vi "set_iterations_per_pixel.vi"(8 "error in (no error)":errorcluster, 10 "iterations per pixel":i32, 11 "FPGAWrapperMH120124FrameScan_PXI7813R in":refnum<class "FPGAWrapperMH120124FrameScan_PXI7813R.lvclass">) -> (0 "error out":errorcluster, 3 "FPGAWrapperMH120124FrameScan_PXI7813R out":refnum<class "FPGAWrapperMH120124FrameScan_PXI7813R.lvclass">)   [LabVIEW 2010, in "FPGAWrapperMH120124FrameScan_PXI7813R.lvclass"]
uses:
  FPGAWrapperMH120124FrameScan_PXI7813R.lvclass
  FPGAWrapperMH120124FrameScan_PXI7813R.lvclass/FPGAWrapperMH120124FrameScan_PXI7813R.ctl
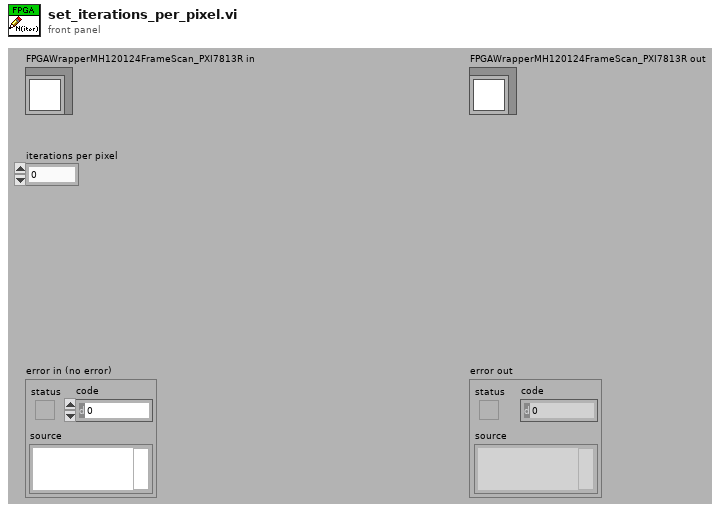
[diagram p1: front panel]
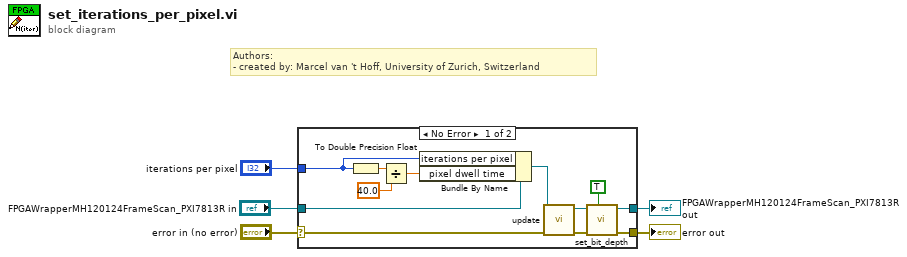
[diagram p0: block diagram]
diagram:
  # "Authors: \n- created by: Marcel van 't Hoff, University of Zurich, Switzerland"
  n1 = case shown="No Error" "error in (no error)" {
    selector: "error in (no error)" -> [w11 w18]
    tunnel: [w6 w18] -> w4
    tunnel: [w7 w19] -> w3
    tunnel: "FPGAWrapperMH120124FrameScan_PXI7813R in" -> [w17 w19]
    tunnel: "iterations per pixel" -> [w13 _]
    frame No Error {
      n2 = To Double Precision Float(number=w13) -> (double precision float=w16:dbl)
      n3 = Divide(x=w16, y=40.0) -> (x/y=w14:dbl)
      n4 = Bundle By Name(cluster=w17, "iterations per pixel"=w13, "pixel dwell time"=w14) -> (w12:refnum<class "FPGAWrapperMH120124FrameScan_PXI7813R.lvclass">)
      n5 = call-dynamic "update.vi"("error in (no error)"=w11, "FPGAWrapperMH120124FrameScan_PXI7813R in"=w12) -> ("error out"=w9:errorcluster, "FPGAWrapperMH120124FrameScan_PXI7813R out"=w8:refnum<class "FPGAWrapperMH120124FrameScan_PXI7813R.lvclass">)  [unwired: 8 in]
      n6 = call-dynamic "set_bit_depth.vi"("calculate by timing? (F)"=TRUE, "error in (no error)"=w9, "FPGAWrapperMH120124FrameScan_PXI7813R in"=w8) -> ("error out"=w6:errorcluster, "FPGAWrapperMH120124FrameScan_PXI7813R out"=w7:refnum<class "FPGAWrapperMH120124FrameScan_PXI7813R.lvclass">)  [unwired: 7 in]
    }
    frame Error {
    }
  }
  "error out" <- w4
  "FPGAWrapperMH120124FrameScan_PXI7813R out" <- w3
